vi "Get DDGIOC Number.vi"(11 "numberPulses":u32) -> (2 "function return":u32, 3 "numberPulses out":u32)   [LabVIEW 2018, in "Copy of Andor SDK.lvlib"]
doc: "EXPNETTYPE unsigned int WINAPI GetDDGIOCNumber(unsigned long * numberPulses);"
uses:
  Copy of Andor SDK.lvlib
  <userlib>/Andor SDK/ATMCD32D.dll
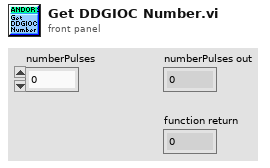
[diagram p1: front panel]
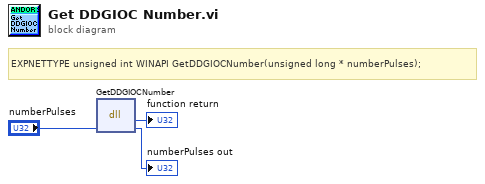
[diagram p0: block diagram]
diagram:
  # "EXPNETTYPE unsigned int WINAPI GetDDGIOCNumber(unsigned long * numberPulses);"
  n1 = dll-call lib="C:/Program Files (x86)/National Instruments/LabVIEW 2018/user.lib/Andor SDK/ATMCD32D.*" fn="GetDDGIOCNumber"("numberPulses"="numberPulses") -> (→"function return":u32, "numberPulses"=→"numberPulses out":u32)  [unwired: 3 in, 2 out]
